vi "Thermometer (Demo).vi"(10 "단위 (0: 섭씨)":u16(ring) items=["섭씨", "화씨"]) -> (1 "온도 값":dbl(slide) scale=0.0..100.0)   [LabVIEW 2015]
doc: "이 VI는 DAQ BNC-2120 터미널 블록의 온도 센서를 사용한 온도 측정을 시뮬레이션합니다.\n\nBNC-2120에 DAQ 보드가 연결되어 있고 MAX로 시스템을 설정한 경우, 이 VI 대신 Thermometer VI를 사용하십시오."
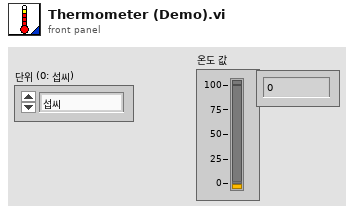
[diagram p1: front panel]
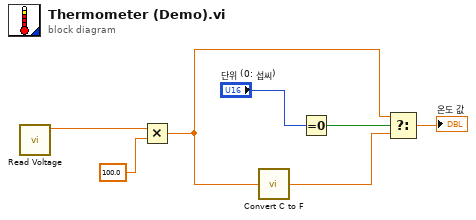
[diagram p0: block diagram]
diagram:
  n1 = call "Read Voltage.vi"() -> ("전압"=w4:dbl)  [unwired: 8 in, 1 out]
  n2 = Multiply(x=w4, y=100.0) -> (x*y=w5:dbl)
  n3 = call "Convert C to F.vi"("섭씨 온도"=w5) -> ("화씨 온도"=w7:dbl)
  n4 = Equal To 0?(x="단위 (0: 섭씨)") -> (x = 0?=w1:bool)
  n5 = Select(t=w5, s=w1, f=w7) -> (s? t:f=→"온도 값":dbl)
